vi "DrawRec.vi"(9 "Color":u32(colorbox)=16711680, 10 "Rectangle":T2, 11 "Image":T1) -> (3 "Image Out":T1)   [LabVIEW 2014]
uses:
  <vilib>/vision/Image Controls.llb/IMAQ Image.ctl
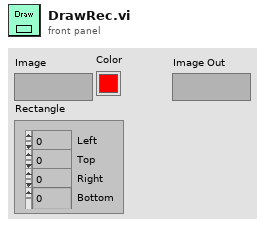
[diagram p1: front panel]
types:
  T1 = typedef "IMAQ Image.ctl" = refnum<image>
  T2 = cluster{"Left":i32, "Top":i32, "Right":i32, "Bottom":i32}
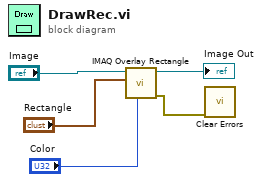
[diagram p0: block diagram]
diagram:
  n1 = call "IMAQ Overlay Rectangle"("Color"="Color", "Rectangle"="Rectangle", "Image"="Image") -> ("error out"=w1:errorcluster, "Image Out"=→"Image Out":T1)  [unwired: 7 in]
  n2 = call <vilib>:"Clear Errors.vi"("error in (no error)"=w1) -> ()  [unwired: 5 in, 2 out]
